vi "XY Graph Set Plots Metadata.vi"(8 "error in (no error)":errorcluster, 9 "Plots Metadata":variant, 11 "XY Graph Refnum":T1) -> (0 "error out":errorcluster, 3 "XY Graph Refnum (dup)":T1)   [LabVIEW 2021, in "XY Graph Add-Ons.lvlib"]
uses:
  XY Graph Add-Ons.lvlib
  XY Graph Refnum.ctl
  XY Graph Property Tag List.ctl
  <vilib>/UserTags/UserTags.lvlib
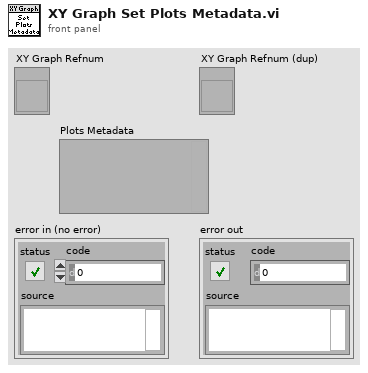
[diagram p1: front panel]
types:
  T1 = typedef "XY Graph Add-Ons.lvlib/XY Graph Refnum.ctl" = refnum<vi>
  T2 = typedef "XY Graph Add-Ons.lvlib/XY Graph Property Tag List.ctl" = enum16{"Max Legend Size", "Preserved Plots", "XScales.GridColors", "YScales.GridColors", "TipStrip String", "TipStrip Visible", "Tool Panels Visibility", "Plots Metadata"}
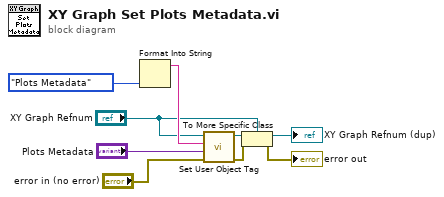
[diagram p0: block diagram]
diagram:
  n1 = Format Into String(XY_Graph_Property_Tag_List."Plots Metadata" ("XY Graph Property Tag")) -> (resulting string=w8:string)  [unwired: 3 in, 1 out]
  n2 = call <vilib>:"Set User Object Tag.vi"("error in (no error)"="error in (no error)", "Value"="Plots Metadata", "Tag Name"=w8, "Generic Refnum"="XY Graph Refnum") -> ("error out"=w4:errorcluster, "dup Generic Refnum"=w6:refnum<vi>)  [unwired: 5 in, 1 out]
  n3 = To More Specific Class(target class="XY Graph Refnum", reference=w6, error in=w4) -> (specific class reference=→"XY Graph Refnum (dup)":T1, error out=→"error out":errorcluster)
